vi "Square root.vi"() -> ()   [LabVIEW 2014]
panel:
  out "Numeric 2":dbl
  in  "Numeric":dbl
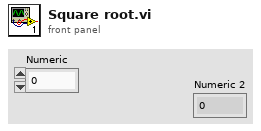
[diagram p1: front panel]
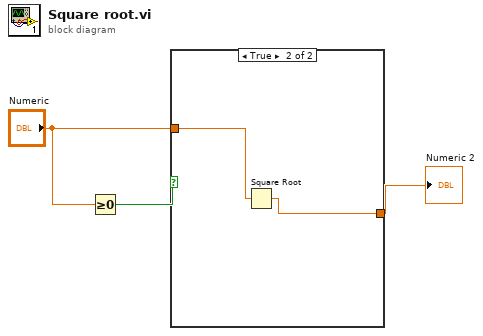
[diagram p0: block diagram]
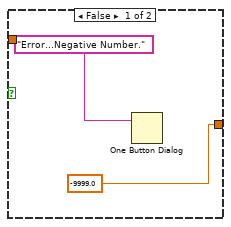
[diagram p2: hidden frame]
diagram:
  n1 = Greater Or Equal To 0?(x="Numeric") -> (x >= 0?=w3:bool)
  n2 = case shown="True" w3 {
    tunnel: "Numeric" -> [_ w7]
    tunnel: [-9999.0 w6] -> w1
    frame False {
      n3 = One Button Dialog(message="Error...Negative Number.") -> ()  [unwired: 1 in, 1 out]
    }
    frame True {
      n4 = Square Root(x=w7) -> (sqrt(x)=w6:dbl)
    }
  }
  "Numeric 2" <- w1
